vi "FA25_FW_pendulum_L3_4_0_oberserve.vi"() -> ()   [LabVIEW 2025]
uses:
  <vilib>/Analysis/Matrix/Datatypes/RealMatrix.ctl
  <vilib>/Analysis/3filter.llb/Filter Passband Type.ctl
  <vilib>/Analysis/baseanly.llb/Real A x B.vi
  <vilib>/Analysis/Matrix/Numeric/Conversions/Array To Matrix - RA2.vi
  <vilib>/Analysis/Matrix/Numeric/Subtract/Subtract - RM,RM.vi
  <vilib>/Analysis/Matrix/Numeric/Conversions/Array To Matrix - RA.vi
  <vilib>/Analysis/Matrix/Numeric/Add/Add - RM,RM.vi
  <vilib>/Analysis/Matrix/Numeric/Multiply/Multiply - RM,R.vi
  <vilib>/Analysis/Matrix/Numeric/Conversions/Matrix To Array - RM.vi
  SADI_Pendulum_lib/pendulumApp.lvlib
  <vilib>/ptbypt/NI_PtbyPt.lvlib
  <vilib>/Analysis/NI_AALBase.lvlib
  <vilib>/Analysis/Matrix/NI_Matrix.lvlib
panel:
  in  "Tab Control":T1(tab)=enum."Plant and Controller"
  out "Firmware Version":sgl=1.002
  out "Software Version":dbl=1.104 format="%_6g"
  out "Number of SADI":i32=1
  out "reset":i32
  out "SADI Connect":i32
  out "P query":i32
  out "P start":i32
  in  "Desired DAQ Loop \nTime (ms)":dbl=0.2
  out "Actual DAQ Loop \nTime (ms)":dbl=0.20860000000084256 format="%#_7g"
  out "Elapsed \nTime (s) daq loop":dbl=15.046546899999953
  out "Txlat_ms":dbl=1.778
  out "min Txlat":dbl=0.682 format="%0.6f"
  out "max TXlat":dbl=4.932 format="%0.6f"
  out "std dev TXlat":dbl=0.7050052541669608 format="%0.6f"
  out "mean  TXlat":dbl=1.2022235999999924 format="%0.6f"
  out "Tx latency, ms":T2(graph)={"X Values"=[0.70325, 0.74575, 0.7882500000000001, 0.8307500000000001, 0.8732500000000001, 0.9157500000000001, 0.95825, 1.00075, 1.04325, 1.0857500000000002, 1.1282500000000002, 1.1707500000000002, 1.2132500000000002, 1.2557500000000001, 1.2982500000000001, 1.34075, 1.38325, 1.42575, 1.46825, 1.51075, 1.55325, 1.59575, 1.63825, 1.68075, 1.72325, 1.76575, 1.8082500000000004, 1.8507500000000003, 1.8932500000000003, 1.9357500000000003, 1.9782500000000003, 2.02075, 2.06325, 2.10575, 2.14825, 2.19075, 2.23325, 2.27575, 2.31825, 2.36075, 2.40325, 2.44575, 2.48825, 2.53075, 2.57325, 2.61575, 2.65825, 2.7007499999999998, 2.7432499999999997, 2.7857499999999997, 2.8282499999999997, 2.8707499999999997, 2.9132499999999997, 2.95575, 2.99825, 3.04075, 3.08325, 3.12575, 3.16825, 3.21075, 3.25325, 3.29575, 3.33825, 3.38075, 3.42325, 3.46575, 3.50825, 3.55075, 3.59325, 3.63575, 3.67825, 3.72075, 3.7632499999999998, 3.8057499999999997, 3.84825, 3.89075, 3.93325, 3.97575, 4.01825, 4.0607500000000005, 4.10325, 4.1457500000000005, 4.18825, 4.2307500000000005, 4.27325, 4.31575, 4.35825, 4.40075, 4.44325, 4.48575, 4.52825, 4.57075, 4.61325, 4.65575, 4.698250000000001, 4.74075, 4.783250000000001, 4.82575, 4.868250000000001, 4.91075], "Histogram: h(x)"=[155, 338, 552, 840, 858, 795, 153, 0, 0, 0, 0, 0, 0, 0, 0, 0, 0, 0, 0, 0, 0, 0, 0, 5, 49, 156, 220, 199, 196, 149, 0, 0, 0, 0, 0, 0, 0, 0, 0, 0, 0, 0, 0, 0, 0, 0, 0, 17, 26, 34, 37, 44, 58, 6, 0, 0, 0, 0, 0, 0, 0, 0, 0, 0, 0, 0, 0, 0, 0, 0, 0, 5, 5, 19, 5, 41, 7, 0, 0, 0, 0, 0, 0, 0, 0, 0, 0, 0, 0, 0, 0, 0, 0, 0, 0, 4, 0, 3, 0, 24]}
  out "ENC VEL":dbl=0.5175486320891765
  out "Pend Rot Error":dbl
  out "Pend Rot Filt":dbl=nan format="%0.2f"
  out "Pendulum velocity":dbl=3.5305560095629e-285
  out "Platen velocity":dbl=0.01738392532814515
  out "Command":dbl=-14.479572053947942
  out "desired\nposition":dbl=-14.790379679306856
  out "Platen Rot Error":dbl format="%0.2f"
  in  "Frequency":dbl=0.5
  in  "Amplitude":dbl=100.0
  in  "Turn On Command":dbl=40.0
  in  "Stop":bool=TRUE
  in  "Desired Loop \nTime (ms)":dbl=1.0
  out "Actual Loop Time (ms)":dbl=1.0000979999995252
  out "Elapsed Time (s)":dbl=15.048252700000035
  out "Segments Saved":u32
  in  "Save Data?":bool
  out "ENC POS":i32=-761
  out "Pendulum ENC":i32
  in  "Sine/Square":bool=TRUE
  in  "Enable Motor":bool=TRUE
  in  "Output Units":enum16{"Degrees", "Radians"}(ring)
  in  "Couts/rev":dbl=3704.0
  in  "Zero":bool
  out "Platen Rotation":dbl=-73.96328293736501
  out "Command Graph":T3(graph)={"Desired Rotation/Command"=-14.479572053947942, -14.479572053947942, 0.0, 0.0}
  out "Desired vs Actual Platen Angle Graph":cluster{"sine wave":dbl, "Filtered x":dbl}(graph)={"sine wave"=-14.479572053947942, "Filtered x"=-73.96328293736501}
  out "Pendulum Rotation Graph":cluster{dbl, dbl}(graph)={nan, 0.0}
  in  "n-int":i32=100
  in  "n-diff":i32=5
  in  "Sampling freq: fs":dbl=1000.0
  in  "Cutoff freq: fl":dbl=10.0 format="%0.3f"
  in  "initialize":bool
  out "PendEncValMax":u16=3687
  out "PendEncValMin":u16=3178
  in  "Pendulum Zero":bool
  out "Pend Rotation":dbl=1440.0 format="%0.2f"
  in  "k":dbl[][](array[numeric])
  out "u":T4
  out "Read Call Error Out":u16(ring)=32768 items=["SADI_RESET (FT_OK)"=0, "FT_INVALID_HANDLE"=1, "FT_DEVICE_NOT_FOUND"=2, "FT_DEVICE_NOT_OPENED"=3, "FT_IO_ERROR"=4, "FT_INSUFFICIENT_RESOURCES"=5, "FT_OTHER_ERROR"=18, "FT_NOT_SUPPORTED"=17, "DATA_RECEIVED"=32768, "NO_DATA_AVAIL"=32769, "NO_SADI"=32770]
  out "SADI State":T5(ring)=enum."Close"
  # "Platen Rotation & Velocity"
  # "Signal Generator"
  # "Butterworth Filter Settings"
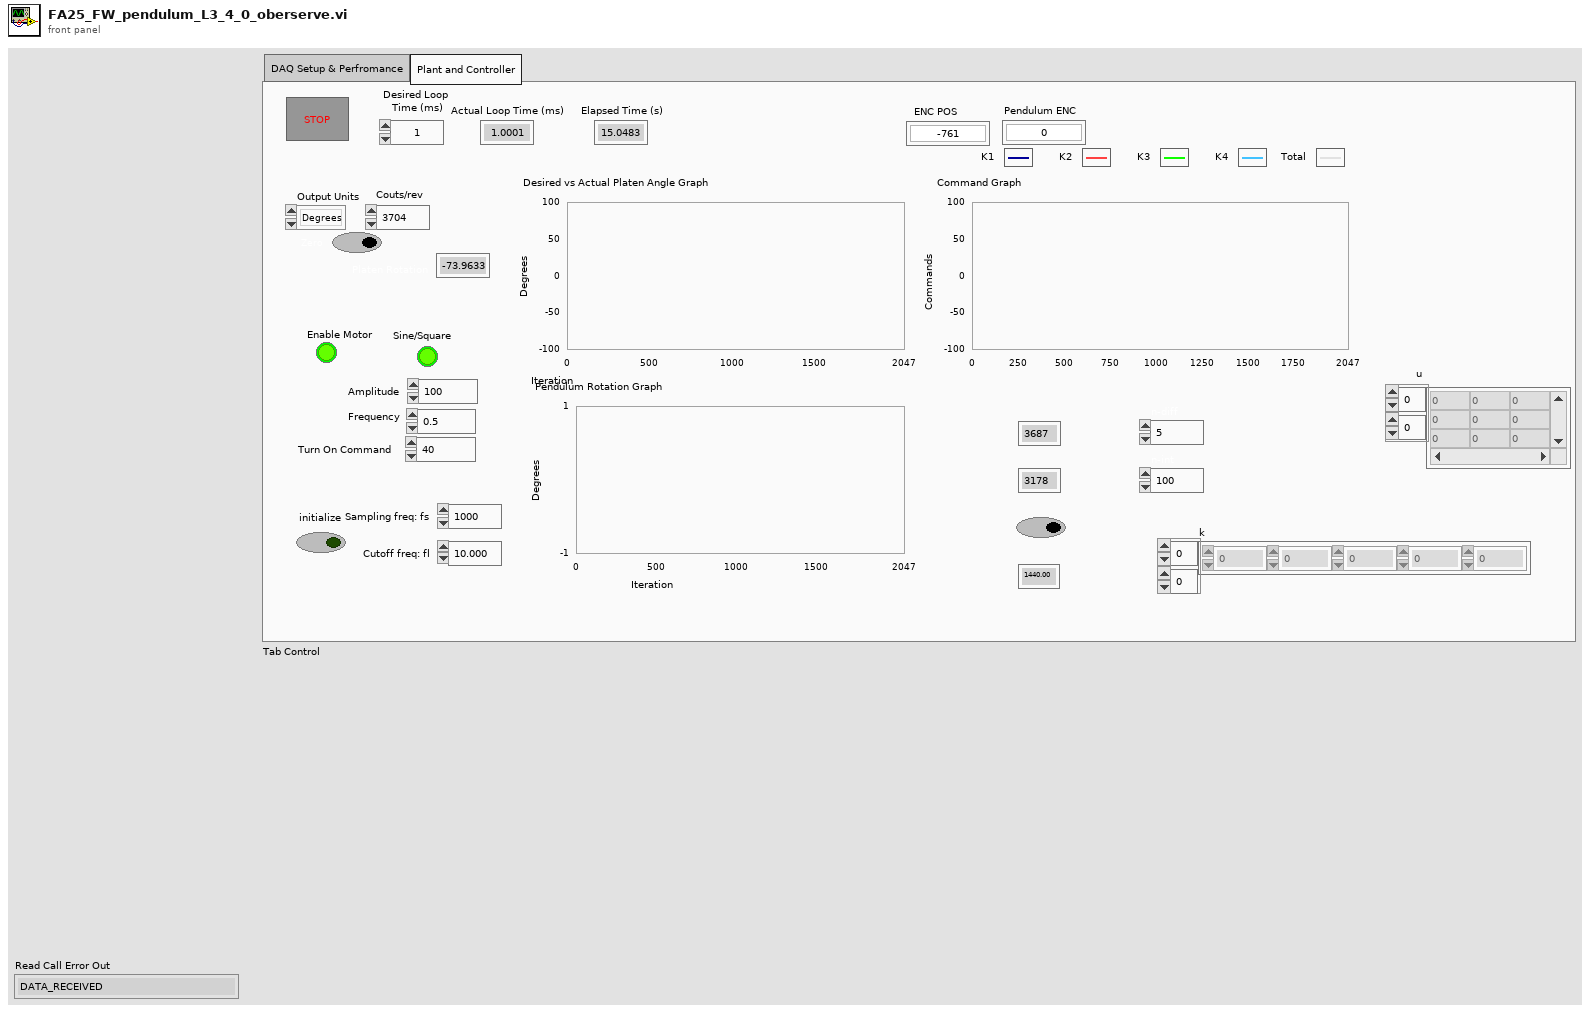
[diagram p1: front panel]
types:
  T1 = enum32{"DAQ Setup & Perfromance", "Plant and Controller"}
  T2 = cluster{"X Values":dbl[], "Histogram: h(x)":i32[]}
  T3 = cluster{"Desired Rotation/Command":dbl, dbl, dbl, dbl}
  T4 = typedef "NI_Matrix.lvlib/RealMatrix.ctl" = dbl[][]
  T5 = enum32{"SADI_check", "Connect_boot", "Check_SW_FW", "Pend_Start", "Run", "Stop", "Store", "Close"}
  T6 = typedef "NI_AALBase.lvlib/Filter Passband Type.ctl" = enum32{"Lowpass", "Highpass", "Bandpass", "Bandstop"}
  T7 = cluster{"desired\nposition":dbl, "Platen Rotation":dbl}
  T8 = cluster{"desired\nposition":dbl, "Command":dbl, dbl, dbl}
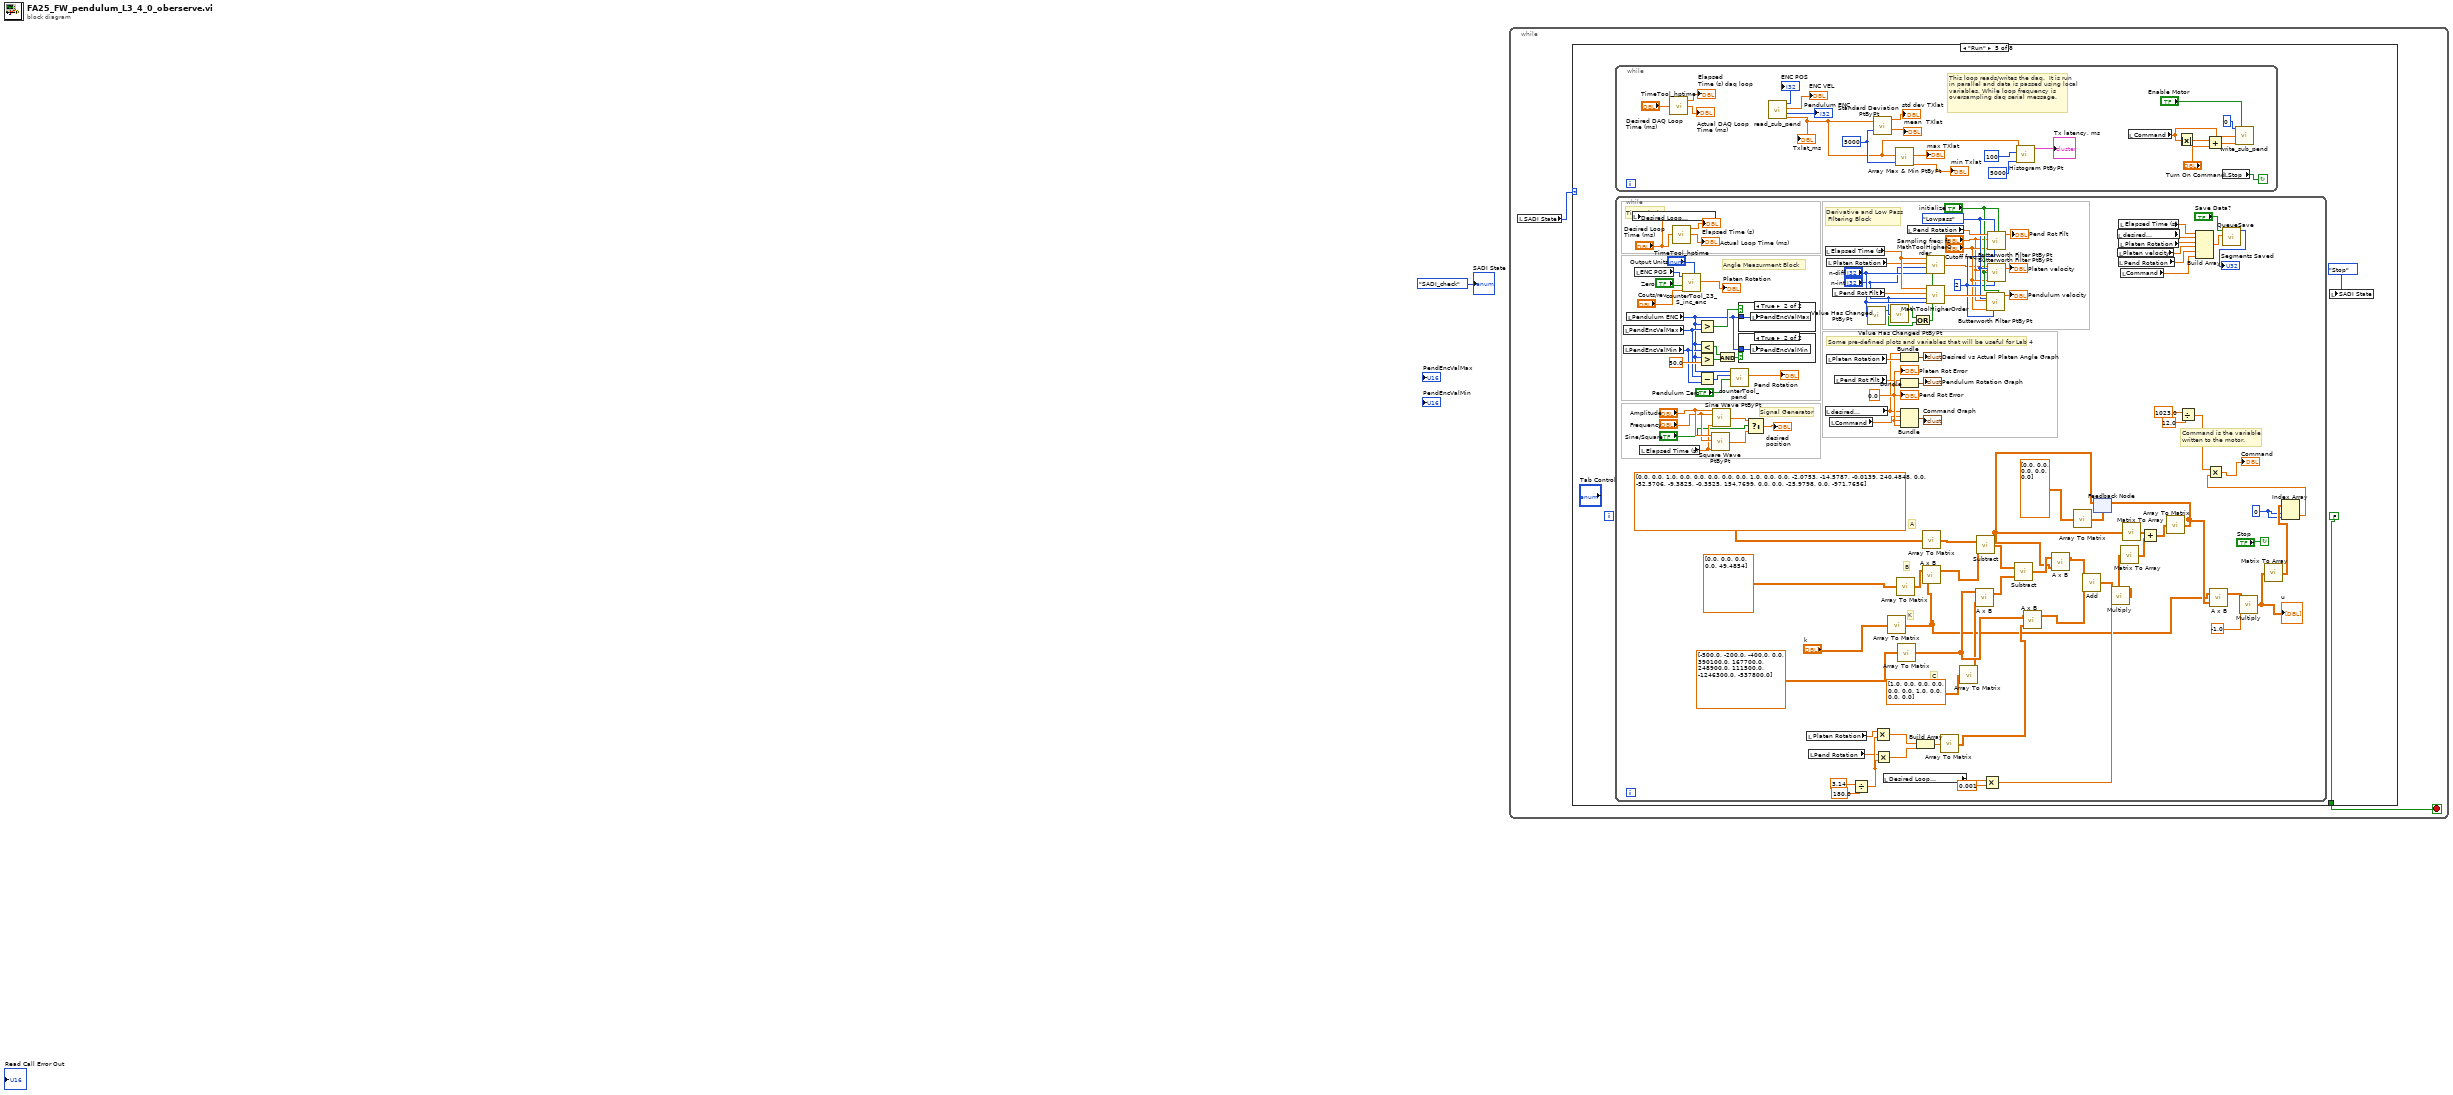
[diagram p0: block diagram]
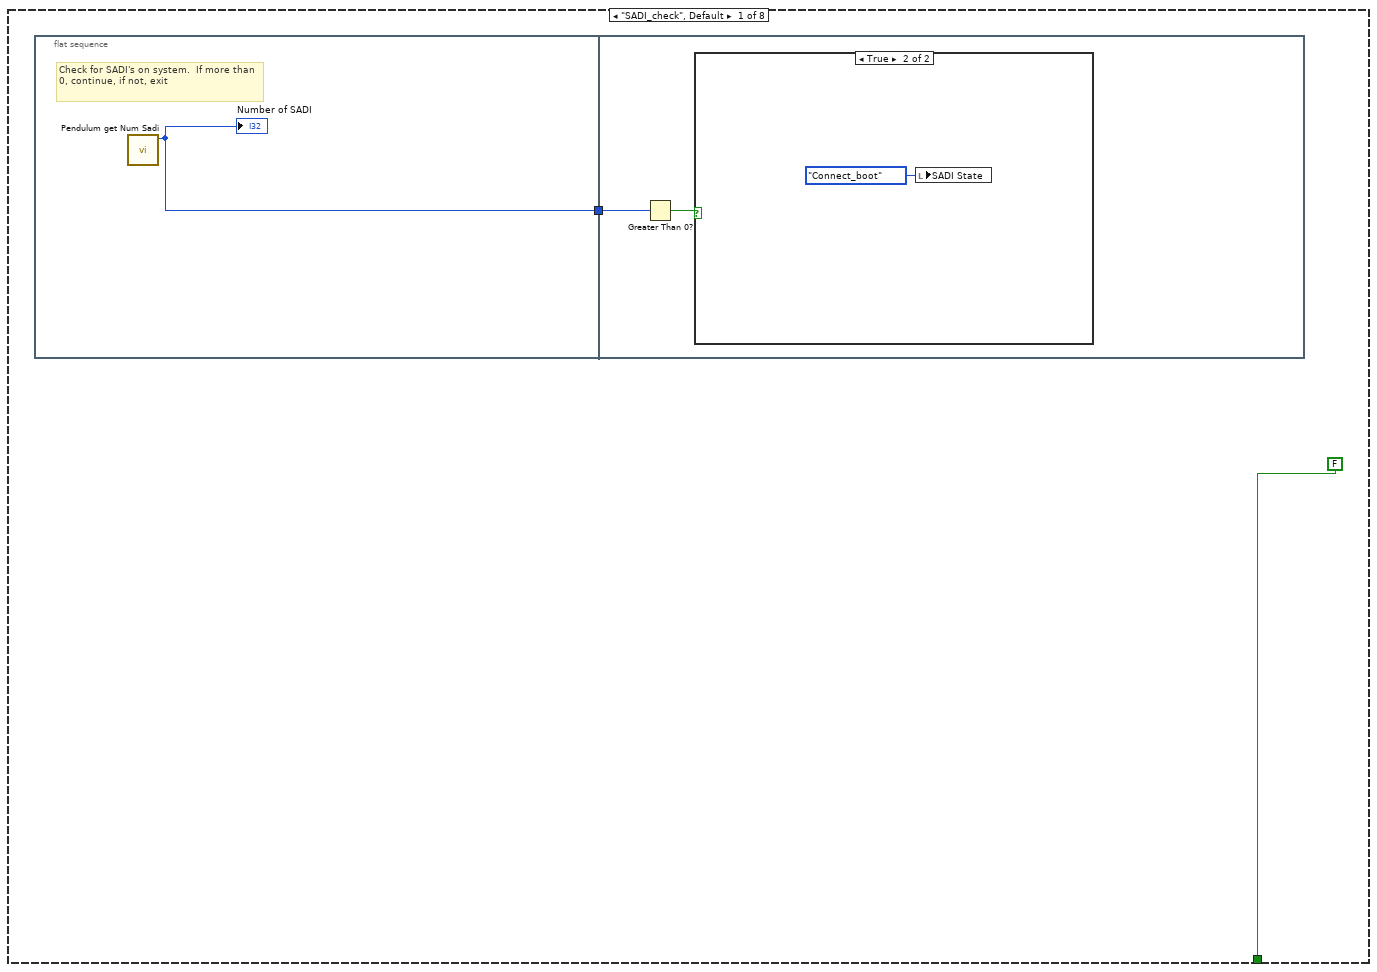
[diagram p2: hidden frame]
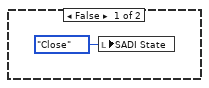
[diagram p3: hidden frame]
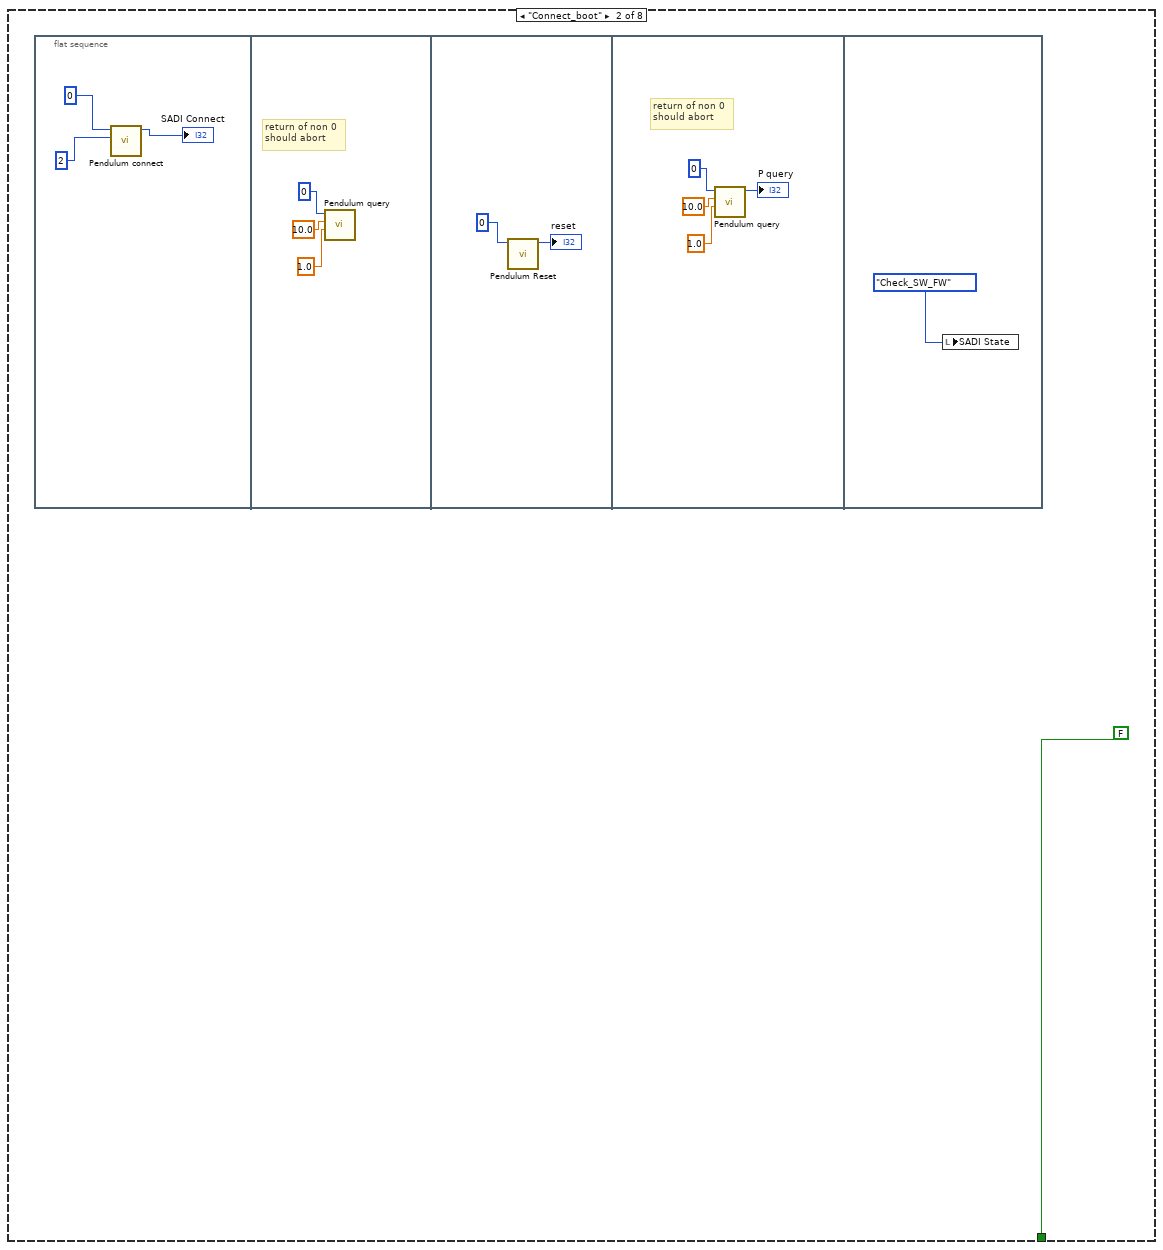
[diagram p4: hidden frame]
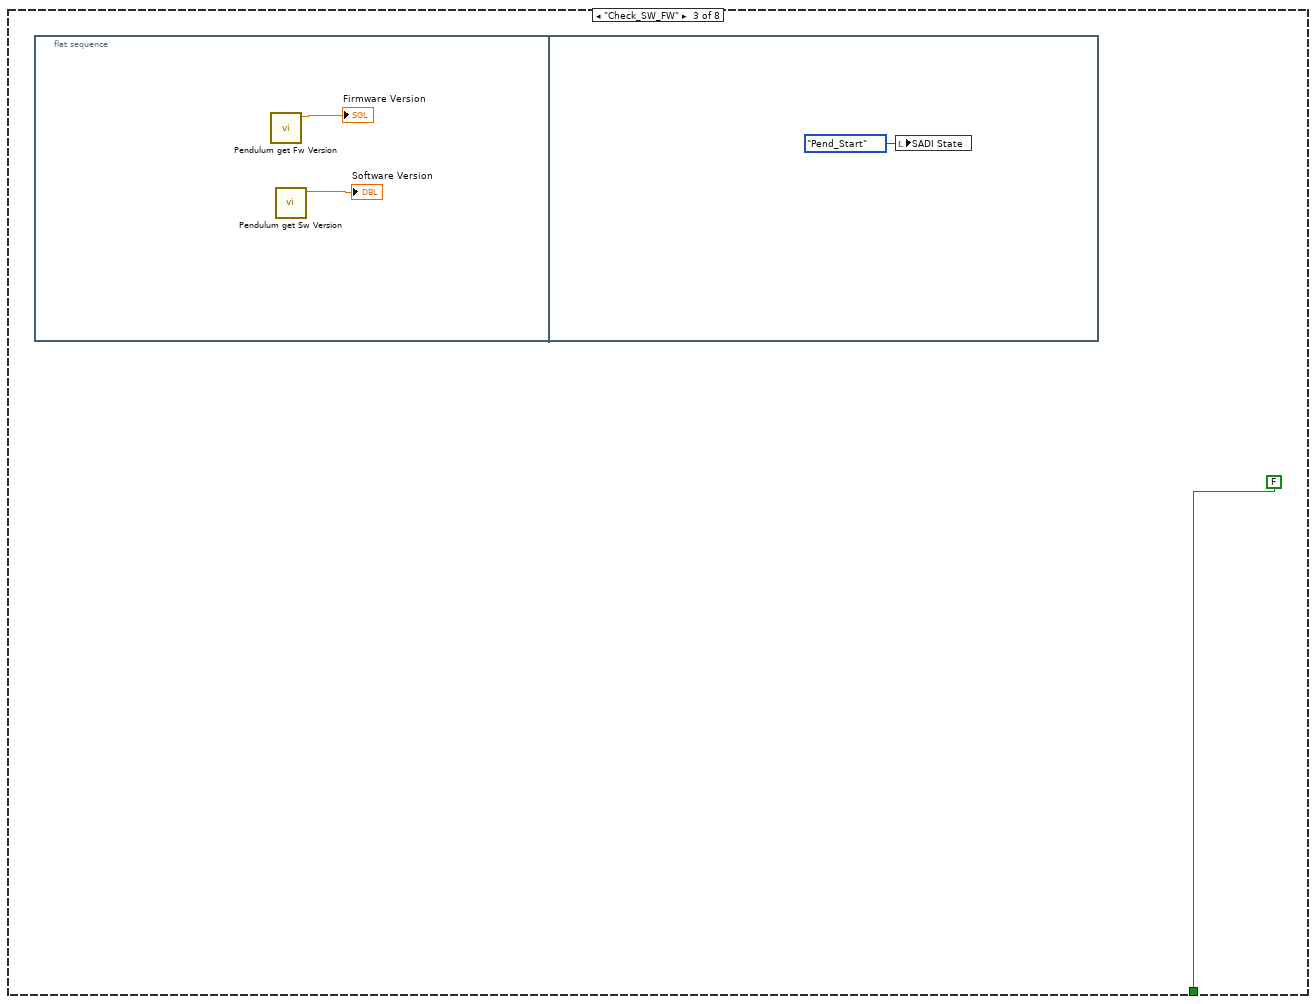
[diagram p5: hidden frame]
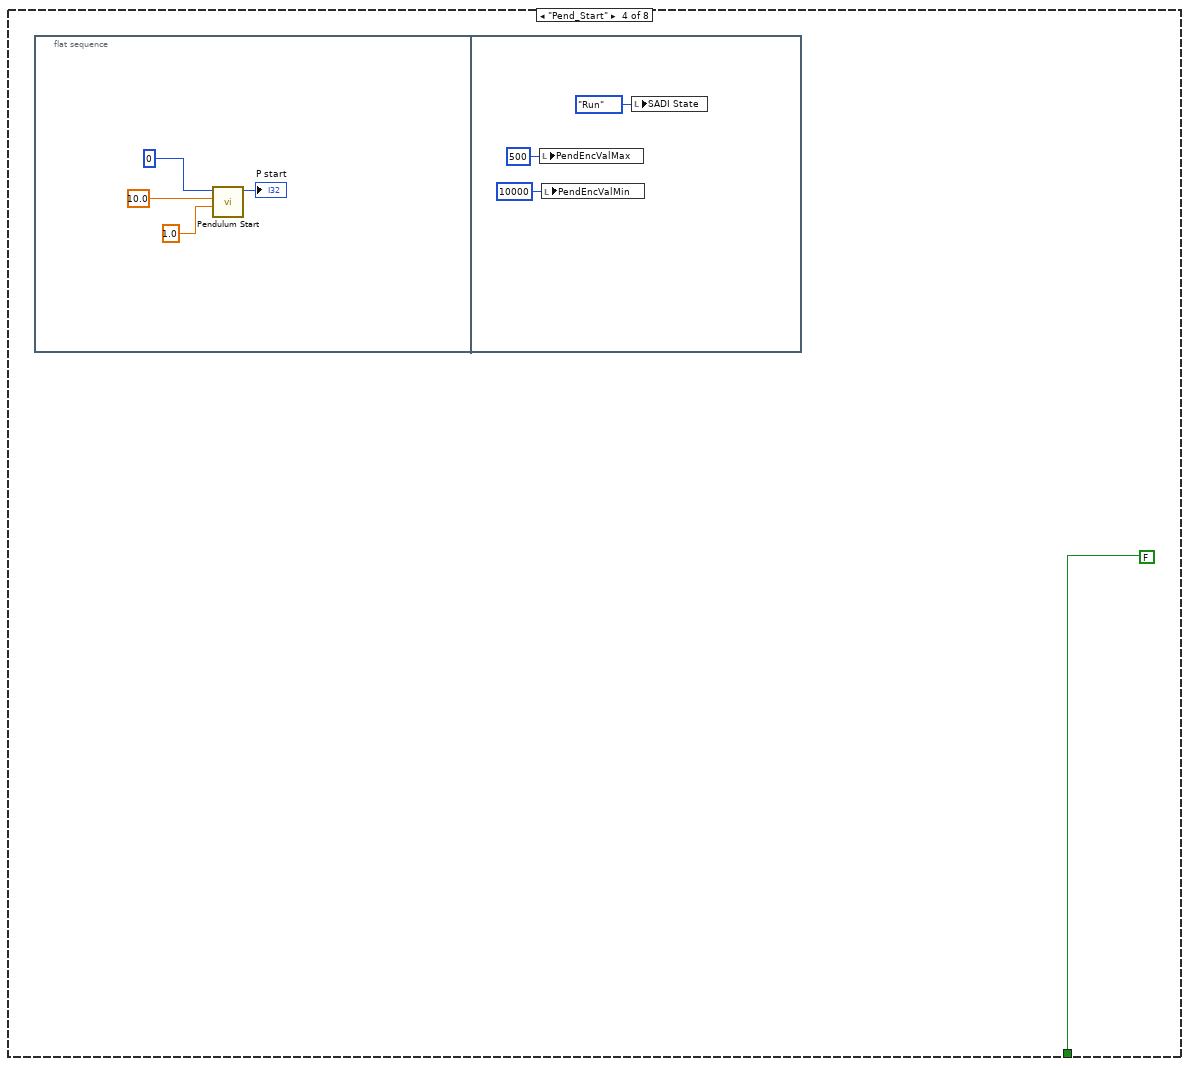
[diagram p6: hidden frame]
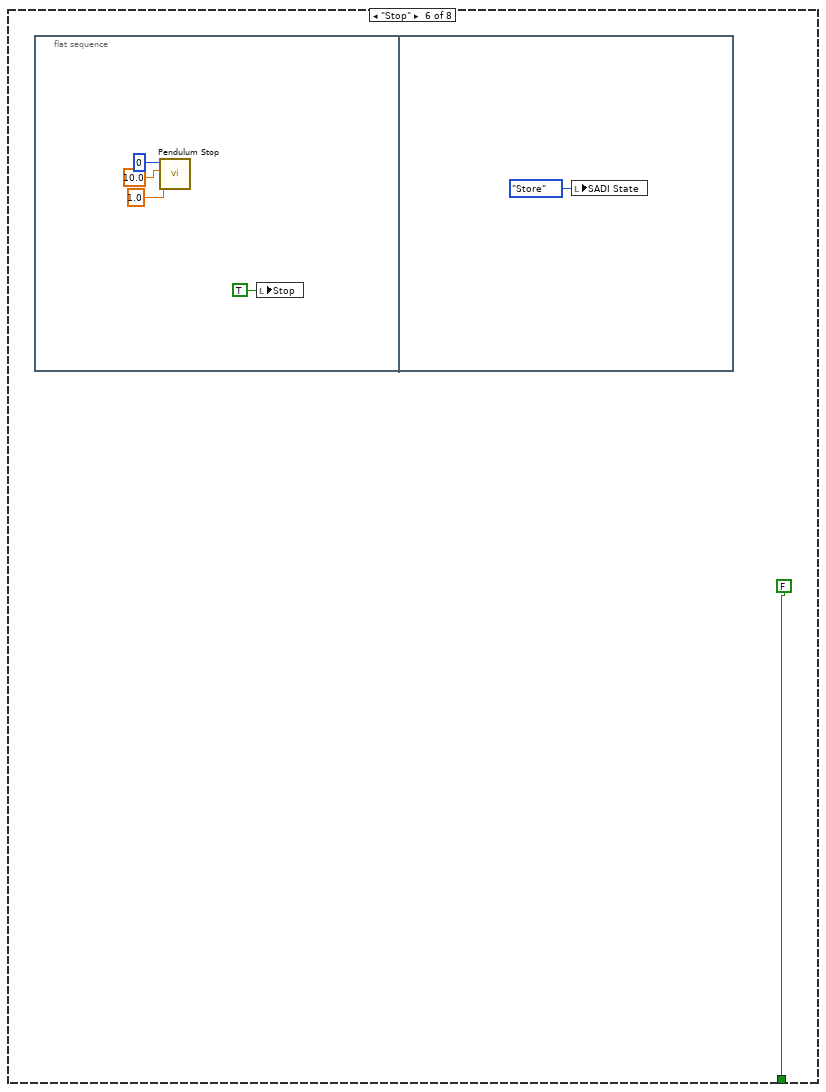
[diagram p9: hidden frame]
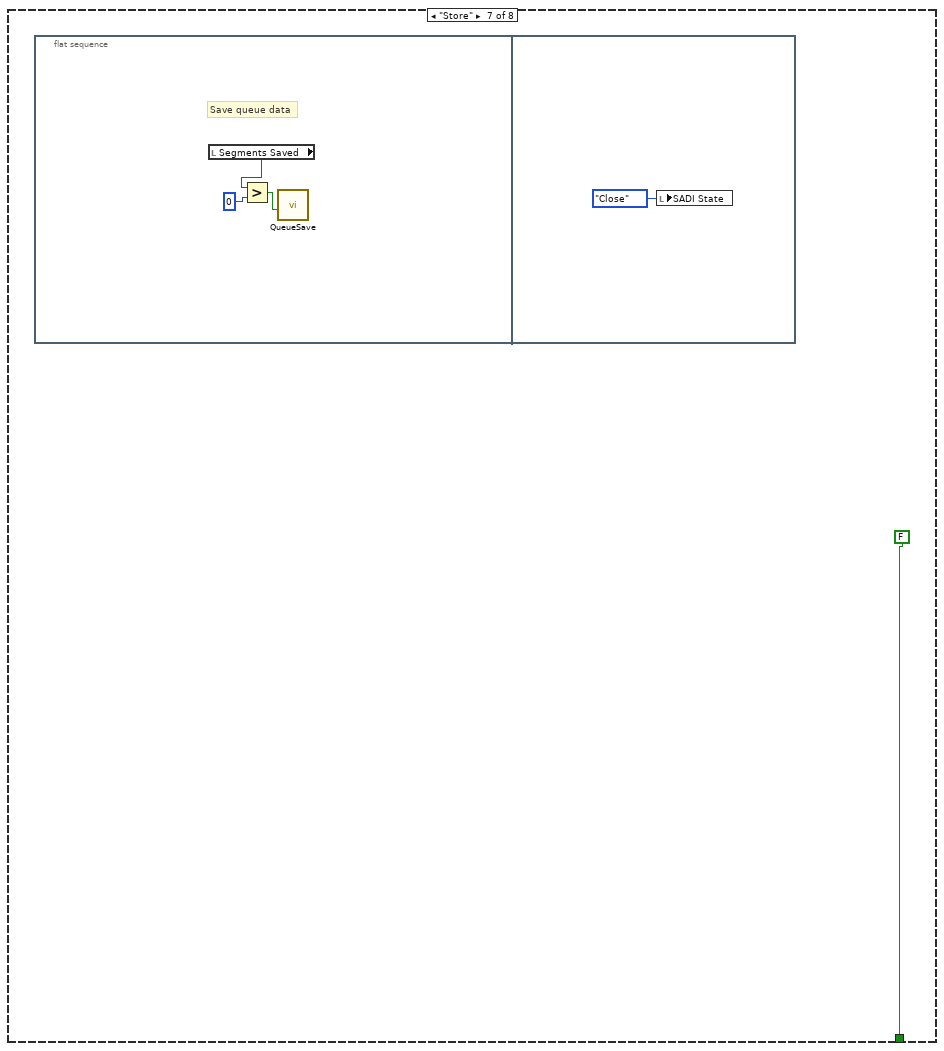
[diagram p10: hidden frame]
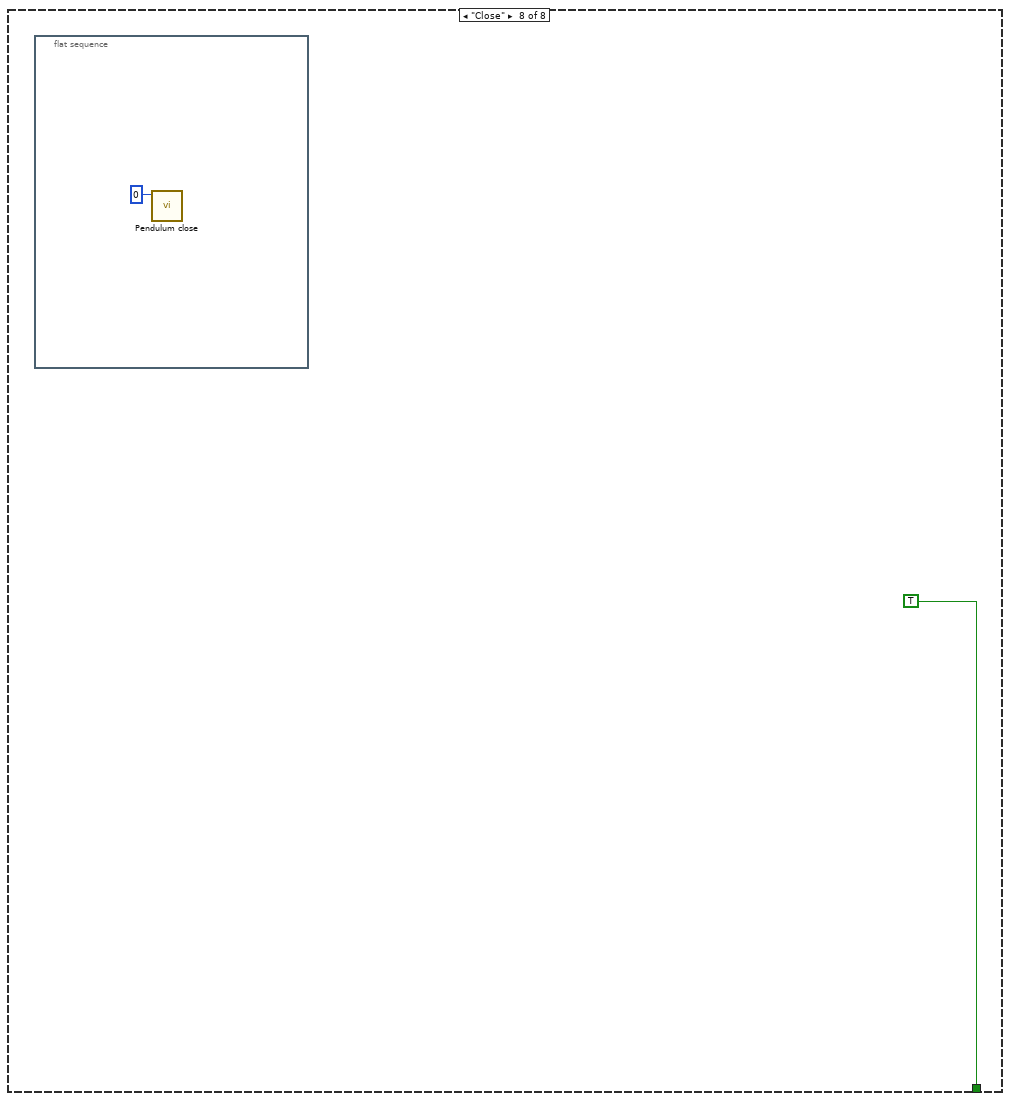
[diagram p11: hidden frame]
diagram:
  n1 = while {
    stop <- w2 stop-if-true
    n2 = local read "SADI State"() -> (w3:T5)
    n3 = case shown="\"Run\"" w3 {
      tunnel: [FALSE FALSE FALSE FALSE FALSE FALSE FALSE TRUE] -> w2
      frame "SADI_check", Default {
        n4 = flat-sequence {
          tunnel: [w6] -> w5
          tunnel: w5 -> [w7]
          frame #0 {
            # "Check for SADI's on system.  If more than 0, continue, if not, exit"
            n5 = call "Pendulum get Num Sadi.vi"() -> ("function return"=w6:i32)  [unwired: 11 in]
            "Number of SADI" <- w6
          }
          frame #1 {
            n6 = Greater Than 0?(x=w7) -> (x > 0?=w8:bool)
            n7 = case shown="True" w8 {
              frame False {
                n8 = local write "SADI State"(T5."Close" ("SADI State")) -> ()
              }
              frame True {
                n9 = local write "SADI State"(T5."Connect_boot" ("SADI State")) -> ()
              }
            }
          }
        }
      }
      frame "Connect_boot" {
        n10 = flat-sequence {
          frame #0 {
            n11 = call "Pendulum connect.vi"("latency_mS"=u8 2, "instance"=0) -> ("function return"=→"SADI Connect":i32)  [unwired: 9 in]
          }
          frame #1 {
            # "return of non 0\nshould abort"
            n12 = call "Pendulum query.vi"("timeout_sec"=1.0, "retry_ms"=10.0, "instance"=0) -> ()  [unwired: 8 in, 1 out]
          }
          frame #2 {
            n13 = call "Pendulum Reset.vi"("instance"=0) -> ("function return"=→"reset":i32)  [unwired: 10 in]
          }
          frame #3 {
            # "return of non 0\nshould abort"
            n14 = call "Pendulum query.vi"("timeout_sec"=1.0, "retry_ms"=10.0, "instance"=0) -> ("function return"=→"P query":i32)  [unwired: 8 in]
          }
          frame #4 {
            n15 = local write "SADI State"(T5."Check_SW_FW" ("SADI State")) -> ()
          }
        }
      }
      frame "Check_SW_FW" {
        n16 = flat-sequence {
          frame #0 {
            n17 = call "Pendulum get Fw Version.vi"() -> ("function return"=→"Firmware Version":dbl)  [unwired: 11 in]
            n18 = call "Pendulum get Sw Version.vi"() -> ("function return"=→"Software Version":dbl)  [unwired: 11 in]
          }
          frame #1 {
            n19 = local write "SADI State"(T5."Pend_Start" ("SADI State")) -> ()
          }
        }
      }
      frame "Pend_Start" {
        n20 = flat-sequence {
          frame #0 {
            n21 = call "Pendulum Start.vi"("timeout_sec"=1.0, "retry_mS"=10.0, "instance"=0) -> ("function return"=→"P start":i32)  [unwired: 8 in]
          }
          frame #1 {
            n22 = local write "PendEncValMax"(u16 500 ("PendEncValMax")) -> ()
            n23 = local write "PendEncValMin"(u16 10000 ("PendEncValMin")) -> ()
            n24 = local write "SADI State"(T5."Run" ("SADI State")) -> ()
          }
        }
      }
      frame "Run" {
        n25 = while {
          stop <- "Stop" continue-if-true
          w62 = 0 ("index (row)")
          w117 = 0.0
          w127 = 2 ("order")
          w129 = Filter_Passband_Type."Lowpass" ("filter type")
          # "C"
          # "L"
          # "K"
          # "B"
          # "A"
          # "Command is the variable \nwritten to the motor."
          # "Some pre-defined plots and variables that will be useful for Lab 4"
          # "Derivative and Low Pass\n FIltering Block"
          # "Angle Measurment Block"
          # "Signal Generator"
          # "Time Block"
          n26 = local read "PendEncValMax"() -> (w143:u16)
          n27 = local read "PendEncValMin"() -> (w142:u16)
          n28 = local read "Pendulum ENC"() -> (w140:i32)
          n29 = local write "Desired Loop \nTime (ms)"("Desired Loop \nTime (ms)") -> ()
          n30 = local read "ENC POS"() -> (w154:i32)
          n31 = local read "Elapsed Time (s)"() -> (w162:dbl)
          n32 = call "TimeTool_hptime.vi"("Desired Loop Time (ms)"="Desired Loop \nTime (ms)") -> ("elapsed time (s)"=→"Elapsed Time (s)":dbl, "dt (ms)"=→"Actual Loop Time (ms)":dbl)  [unwired: 1 out]
          n33 = call "counterTool_23_S_inc_enc.vi"("Counts"=w154, "Zero"="Zero", "Couts/rev"="Couts/rev", "Output Units"="Output Units") -> ("Total Angle"=→"Platen Rotation":dbl)  [unwired: 3 in, 1 out]
          n34 = Greater?(x=w140, y=w143) -> (0:w147:bool)
          n35 = Less?(x=w140, y=w142) -> (x < y?=w149:bool)
          n36 = Greater?(x=w140, y=50.0) -> (0:w148:bool)
          n37 = Subtract(x=w143, y=w142) -> (x-y=w144:u16)
          n38 = call <vilib>:"Square Wave PtByPt.vi"("amplitude"="Amplitude", "frequency"="Frequency", "time"=w162) -> ("square wave"=w159:dbl)  [unwired: 2 in]
          n39 = call <vilib>:"Sine Wave PtByPt.vi"("time"=w162, "frequency"="Frequency", "amplitude"="Amplitude") -> ("sine wave"=w160:dbl)  [unwired: 1 in]
          n40 = And(x=w149, y=w148) -> (x .and. y?=w146:bool)
          n41 = call "counterTool_pend.vi"("Counts"=w140, "Pendulum Scale"=w144, "Zero"="Pendulum Zero") -> ("Total Angle"=→"Pend Rotation":dbl)  [unwired: 4 in, 1 out]
          n42 = case shown="True" w147 {
            tunnel: w140 -> [_ w172]
            frame False {
            }
            frame True {
              n43 = local write "PendEncValMax"(w172) -> ()
            }
          }
          n44 = case shown="True" w146 {
            tunnel: w140 -> [_ w171]
            frame False {
            }
            frame True {
              n45 = local write "PendEncValMin"(w171) -> ()
            }
          }
          n46 = Select(t=w160, s="Sine/Square", f=w159) -> (s? t:f=→"desired\nposition":dbl)
          n47 = local read "Platen Rotation"() -> (w99:dbl)
          n48 = local read "Pend Rotation"() -> (w98:dbl)
          n49 = local read "Elapsed Time (s)"() -> (w138:dbl)
          n50 = local read "desired\nposition"() -> (w110:dbl)
          n51 = local read "Platen Rotation"() -> (w116:dbl)
          n52 = local read "Platen Rotation"() -> (w133:dbl)
          n53 = local read "Command"() -> (w109:dbl)
          n54 = local read "Pend Rot Filt"() -> (w132:dbl)
          n55 = local read "Pend Rot Filt"() -> (w115:dbl)
          n56 = Divide(x=3.14, y=180.0) -> (x/y=w100:dbl)
          n57 = call <vilib>:"Value Has Changed PtByPt.vi"("input data point"="n-diff") -> ("has changed"=w121:bool)  [unwired: 1 in, 1 out]
          n58 = Multiply(x=w99, y=w100) -> (x*y=w96:dbl)
          n59 = Multiply(x=w98, y=w100) -> (x*y=w97:dbl)
          n60 = local read "Desired Loop \nTime (ms)"() -> (w94:dbl)
          n61 = call-poly <vilib>:"Array To Matrix.vi"("Real 2D Array"="k") -> ("Real Matrix"=w67:T4)
          n62 = call <vilib>:"Value Has Changed PtByPt.vi"("input data point"="n-int") -> ("has changed"=w122:bool)  [unwired: 1 in, 1 out]
          n63 = call-poly <vilib>:"Array To Matrix.vi"("Real 2D Array"=dbl[][] [[0.0], [0.0], [0.0], [0.0], [49.4854]] ("x")) -> ("Real Matrix"=w75:T4)
          n64 = call-poly <vilib>:"Array To Matrix.vi"("Real 2D Array"=dbl[][] [[-500.0, -200.0], [-400.0, 0.0], [390100.0, 167700.0], [248900.0, 111500.0], [-1246300.0, -537800.0]] ("x")) -> ("Real Matrix"=w78:T4)
          n65 = Bundle("desired\nposition"=w110, "Platen Rotation"=w116) -> (→"Desired vs Actual Platen Angle Graph":T7)  [unwired: 1 in]
          n66 = Bundle("Pend Rot Filt"=w115, w117) -> (→"Pendulum Rotation Graph":cluster{"Pend Rot Filt":dbl, dbl})  [unwired: 1 in]
          n67 = Bundle("desired\nposition"=w110, "Command"=w109, w117, w117) -> (→"Command Graph":T8)  [unwired: 1 in]
          n68 = local read "Pend Rotation"() -> (w134:dbl)
          n69 = Or(x=w122, y=w121) -> (x .or. y?=w136:bool)
          n70 = Build Array(w96, w97) -> (w95:dbl[])
          n71 = call-poly <vilib>:"A x B.vi"("B"=w67, "A"=w75) -> ("A x B"=w76:T4)  [unwired: 1 out]
          n72 = call-poly <vilib>:"Array To Matrix.vi"("Real 2D Array"=dbl[][] [[0.0, 0.0, 1.0, 0.0, 0.0], [0.0, 0.0, 0.0, 1.0, 0.0], [0.0, -2.0753, -14.5787, -0.0139, 240.4848], [0.0, -52.5706, -9.3825, -0.3525, 154.7699], [0.0, 0.0, -25.9798, 0.0, -971.7656]]) -> ("Real Matrix"=w90:T4)
          n73 = call "MathToolHigherOrder.vi"("Time"=w138, "Data"=w133, "n-int"="n-int", "Reset (F)"=w136, "n-diff"="n-diff") -> ("1st derivative"=w123:dbl)  [unwired: 1 in, 2 out]
          n74 = call "MathToolHigherOrder.vi"("Time"=w138, "Data"=w132, "n-int"="n-int", "Reset (F)"=w136, "n-diff"="n-diff") -> ("1st derivative"=w130:dbl)  [unwired: 1 in, 2 out]
          n75 = call-poly <vilib>:"Array To Matrix.vi"("Real 1D Array"=w95) -> ("Real Matrix (Column Vector)"=w80:T4)
          n76 = call-poly <vilib>:"Array To Matrix.vi"("Real 2D Array"=dbl[][] [[1.0, 0.0, 0.0, 0.0, 0.0], [0.0, 1.0, 0.0, 0.0, 0.0]] ("y")) -> ("Real Matrix"=w77:T4)
          n77 = call-poly <vilib>:"A x B.vi"("B"=w77, "A"=w78) -> ("A x B"=w79:T4)  [unwired: 1 out]
          n78 = call-poly <vilib>:"Subtract.vi"("Real Matrix B"=w76, "Real Matrix A"=w90) -> ("A - B"=w103:T4)
          n79 = Multiply(x=w94, y=0.001) -> (x*y=w91:dbl)
          n80 = call <vilib>:"Butterworth Filter PtByPt.vi"("initialize"="initialize", "order"=w127, "filter type"=w129, "low cutoff freq: fl"="Cutoff freq: fl", "sampling freq: fs"="Sampling freq: fs", "x"=w130) -> ("Filtered x"=→"Pendulum velocity":dbl)  [unwired: 3 in, 1 out]
          n81 = call <vilib>:"Butterworth Filter PtByPt.vi"("initialize"="initialize", "order"=w127, "filter type"=w129, "low cutoff freq: fl"="Cutoff freq: fl", "sampling freq: fs"="Sampling freq: fs", "x"=w134) -> ("Filtered x"=→"Pend Rot Filt":dbl)  [unwired: 3 in, 1 out]
          n82 = call <vilib>:"Butterworth Filter PtByPt.vi"("initialize"="initialize", "order"=w127, "filter type"=w129, "low cutoff freq: fl"="Cutoff freq: fl", "sampling freq: fs"="Sampling freq: fs", "x"=w123) -> ("Filtered x"=→"Platen velocity":dbl)  [unwired: 3 in, 1 out]
          n83 = call-poly <vilib>:"Subtract.vi"("Real Matrix B"=w79, "Real Matrix A"=w103) -> ("A - B"=w82:T4)
          n84 = call-poly <vilib>:"A x B.vi"("B"=w80, "A"=w78) -> ("A x B"=w81:T4)  [unwired: 1 out]
          n85 = call-poly <vilib>:"Array To Matrix.vi"("Real 2D Array"=dbl[][] [[0.0], [0.0], [0.0], [0.0], [0.0]]) -> ("Real Matrix"=w74:T4)
          n86 = feedback #1(w74) -> (w72:T4)
          n87 = call-poly <vilib>:"A x B.vi"("B"=w72, "A"=w82) -> ("A x B"=w83:T4)  [unwired: 1 out]
          n88 = call-poly <vilib>:"Add.vi"("Real Matrix B"=w81, "Real Matrix A"=w83) -> ("A + B"=w92:T4)
          n89 = call-poly <vilib>:"Multiply.vi"("Real Scalar c"=w91, "Real Matrix A"=w92) -> ("A * c"=w71:T4)
          n90 = local read "desired\nposition"() -> (w151:dbl)
          n91 = local read "Platen velocity"() -> (w113:dbl)
          n92 = local read "Pend Rotation"() -> (w112:dbl)
          n93 = local read "Elapsed Time (s)"() -> (w169:dbl)
          n94 = local read "Platen Rotation"() -> (w114:dbl)
          n95 = local read "Command"() -> (w111:dbl)
          n96 = call-poly <vilib>:"Matrix To Array.vi"("Real Matrix"=w71) -> ("Real 2D Array"=w70:dbl[][])
          n97 = call-poly <vilib>:"Matrix To Array.vi"("Real Matrix"=w72) -> ("Real 2D Array"=w69:dbl[][])
          n98 = Add ("Add.vi")(x=w69, y=w70) -> (x+y=w73:dbl[][])
          n99 = call-poly <vilib>:"Array To Matrix.vi"("Real 2D Array"=w73) -> ("Real Matrix"=w68:T4)
          n100 = feedback-in #1(w68) -> ()
          n101 = Divide(x=1023.0, y=12.0) -> (x/y=w107:dbl)
          n102 = Build Array(w169, w151, w114, w113, w112, w111) -> (w168:dbl[])
          n103 = call-poly <vilib>:"A x B.vi"("B"=w68, "A"=w67) -> ("A x B"=w66:T4)  [unwired: 1 out]
          n104 = call "QueueSave.vi"("Data In"=w168, "Save Data?"="Save Data?") -> ("Segments Saved"=→"Segments Saved":u32)  [unwired: 3 in, 2 out]
          n105 = call-poly <vilib>:"Multiply.vi"("Real Scalar c"=-1.0, "Real Matrix A"=w66) -> ("A * c"=w64:T4)
          "u" <- w64
          n106 = call-poly <vilib>:"Matrix To Array.vi"("Real Matrix"=w64) -> ("Real 2D Array"=w63:dbl[][])
          n107 = Index Array(array=w63, index (row)=w62, index (col)=w62) -> (element=w61:dbl)
          n108 = Multiply(x=w107, y=w61) -> (x*y=→"Command":dbl)
          "Platen Rot Error" <- w117
          "Pend Rot Error" <- w117
        }
        n109 = while {
          stop <- w40 continue-if-true
          w54 = 5000 ("sample length")
          # "This loop reads/writes the daq.  It is run in parallel and data is passed using local variables. While loop frequency is oversampling daq serial message."
          n110 = call "TimeTool_hptime.vi"("Desired Loop Time (ms)"="Desired DAQ Loop \nTime (ms)") -> ("elapsed time (s)"=→"Elapsed \nTime (s) daq loop":dbl, "dt (ms)"=→"Actual DAQ Loop \nTime (ms)":dbl)  [unwired: 1 out]
          n111 = call "read_sub_pend.vi"() -> ("Txlat_ms"=w49:dbl, "Pendulum ENC 2"=→"Pendulum ENC":i32, "ENC VEL 1"=→"ENC VEL":dbl, "ENC POS 1"=→"ENC POS":i32)  [unwired: 7 in]
          "Txlat_ms" <- w49
          n112 = call <vilib>:"Standard Deviation PtByPt.vi"("x"=w49, "sample length"=w54) -> ("standard deviation"=→"std dev TXlat":dbl, "mean"=→"mean  TXlat":dbl)  [unwired: 1 in, 1 out]
          n113 = call <vilib>:"Array Max & Min PtByPt.vi"("input data point"=w49, "sample length"=w54) -> ("max value"=→"max TXlat":dbl, "min value"=→"min Txlat":dbl)  [unwired: 1 in, 3 out]
          n114 = call <vilib>:"Histogram PtByPt.vi"("sample length"=5000, "intervals"=100, "x"=w49) -> ("Histogram Graph"=→"Tx latency, ms":T2)  [unwired: 5 in, 3 out]
          n115 = local read "Command"() -> (w39:dbl)
          n116 = Absolute Value(x=w39) -> (abs(x)=w45:dbl)
          n117 = Add(x=w45, y="Turn On Command") -> (x+y=w46:dbl)
          n118 = local read "Stop"() -> (w40:bool)
          n119 = call "write_sub_pend.vi"("instance"=0, "Enable Motor"="Enable Motor", "direction"=w39, "motorEffort"=w46) -> ()  [unwired: 12 in]
        }
        n120 = local write "SADI State"(T5."Stop" ("SADI State")) -> ()
      }
      frame "Stop" {
        n121 = flat-sequence {
          frame #0 {
            n122 = call "Pendulum Stop.vi"("timeout_sec"=1.0, "retry_mS"=10.0, "instance"=0) -> ()  [unwired: 8 in, 1 out]
            n123 = local write "Stop"(TRUE ("Stop")) -> ()
          }
          frame #1 {
            n124 = local write "SADI State"(T5."Store" ("SADI State")) -> ()
          }
        }
      }
      frame "Store" {
        n125 = flat-sequence {
          frame #0 {
            # "Save queue data"
            n126 = local read "Segments Saved"() -> (w182:u32)
            n127 = Greater?(x=w182, y=u32 0) -> (0:w181:bool)
            n128 = call "QueueSave.vi"("Write To Spreadsheet"=w181) -> ()  [unwired: 4 in, 3 out]
          }
          frame #1 {
            n129 = local write "SADI State"(T5."Close" ("SADI State")) -> ()
          }
        }
      }
      frame "Close" {
        n130 = flat-sequence {
          frame #0 {
            n131 = call "Pendulum close.vi"("instance"=0) -> ()  [unwired: 10 in, 1 out]
          }
        }
      }
    }
  }
  "SADI State" <- T5."SADI_check" ("SADI State")
